vi "SUB_Delay ms.vi"(3 "delay(ms)":u32) -> ()   [LabVIEW 2015]
doc: "GUID stands for <B>G</B>lobally <B>U</B>nique <B>ID</B>entifier, a 128-bit integer used as unique identifier.\n\nThis VI makes a call to ole32.dll to create an absolutely unique number that you can use as a persistent identifier in a distributed environment.To a very high degree of certainty, this function returns a unique value: no other invocation, on the same or any other system (networked or not), should return the same value.\n\n<B>GUID Cluster</B> returns the GUID in a cluster that follows the GUID format.\n\n<B>GUID String</B> has the GUID as a string of characters.\n\n<B>GUID OLE String</B> has a format like that of the following sample:\n\n{c200e360-38c5-11ce-ae62-08002b2b79ef} \n \nwhere the successive fields break the GUID into the form:\n\nDWORD-WORD-WORD-WORD-WORD-DWORD\n\ncovering the 128-bit GUID. The string includes the enclosing braces, which are an OLE convention.\n\nEnrique Vargas\nvargas@jyestudio.com"
panel:
  out "time(ms)":u32
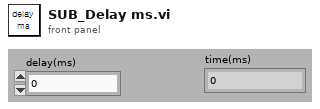
[diagram p1: front panel]
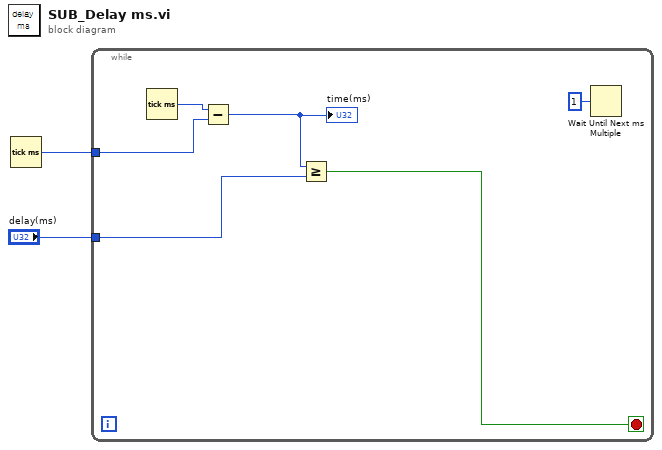
[diagram p0: block diagram]
diagram:
  n1 = Tick Count (ms)() -> (millisecond timer value=w2:u32)
  n2 = while {
    tunnel: w2 -> [w6]
    tunnel: "delay(ms)" -> [w4]
    stop <- w3 stop-if-true
    n3 = Tick Count (ms)() -> (millisecond timer value=w7:u32)
    n4 = Subtract(x=w7, y=w6) -> (x-y=w5:u32)
    "time(ms)" <- w5
    n5 = Greater Or Equal?(x=w5, y=w4) -> (x >= y?=w3:bool)
    n6 = Wait Until Next ms Multiple(millisecond multiple=u32 1 ("ms 배수")) -> ()  [unwired: 1 out]
  }
